vi "Add Boost Stage.vi"(8 "error in (no error)":errorcluster, 10 "Stage Name":string, 11 "Shot Section Item Ref":T1=18446744073709551615 format="%.0x") -> (0 "error out":errorcluster, 3 "Shot Section Item Ref dup":T1=18446744073709551615 format="%.0x")   [LabVIEW 2019, in "Fuel Injector Analysis Addon System Explorer.lvlib"]
uses:
  Fuel Injector Analysis Addon System Explorer.lvlib
  <vilib>/NI VeriStand/Custom Device API/Custom Device Item Ref.ctl
  Addon Shared/Types/Analysis.Channels.Select.ctl
  Addon Shared/Constants.vi
  Addon Shared/Fuel Injector Analysis Addon Shared.lvlib
  <vilib>/NI VeriStand/Custom Device API/Custom Device API.lvlib
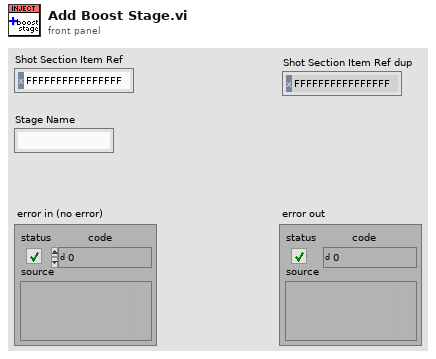
[diagram p1: front panel]
types:
  T1 = typedef "Custom Device API.lvlib/Custom Device Item Ref.ctl" = u64
  T2 = typedef "Fuel Injector Analysis Addon Shared.lvlib/Analysis.Channels.Select.ctl" = cluster{"Pull In Time":bool, "Pull In Max Current":bool, "Pull In Max Voltage":bool, "Pull In Min Voltage":bool, "Pull In Avg Voltage":bool, "Hold Time":bool, "Hold Max Current":bool, "Hold Min Current":bool, "Hold Avg Current":bool, "Hold Max Voltage":bool, "Hold Min Voltage":bool, "Hold Avg Max Voltage":bool, "Hold Avg Min Voltage":bool, "Off Time":bool, "Off Max Current":bool, "Off Min Current":bool, "Off Avg Current":bool, "Off Max Voltage":bool, "Off Min Voltage":bool, "Off Avg Voltage":bool, "Total Voltage Pulses":bool, "Total Stage Time":bool}
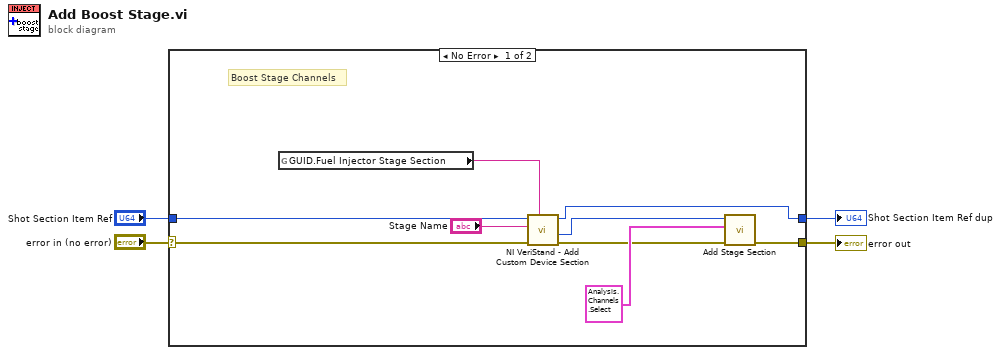
[diagram p0: block diagram]
diagram:
  n1 = case shown="No Error" "error in (no error)" {
    selector: "error in (no error)" -> [w11 w14]
    tunnel: "Shot Section Item Ref" -> [w10 w15]
    tunnel: [w5 w15] -> w2
    tunnel: [w13 w14] -> w1
    frame No Error {
      # "Boost Stage Channels"
      n2 = global read "Constants.vi" "GUID.Fuel Injector Stage Section"() -> (w12:string)
      n3 = call <vilib>:"NI VeriStand - Add Custom Device Section.vi"("GUID (Default Section)"=w12, "error in (no error)"=w11, "Section Name"="Stage Name", "Parent Ref in"=w10) -> ("error out"=w7:errorcluster, "Section Ptr"=w6:T1, "Parent Ref out"=w5:T1)  [unwired: 4 in, 1 out]
      n4 = call "Add Stage Section.vi"("error in (no error)"=w7, "Analysis Options"=T2 {"Pull In Time"=TRUE, "Pull In Max Current"=TRUE, "Pull In Max Voltage"=TRUE, "Pull In Min Voltage"=TRUE, "Pull In Avg Voltage"=TRUE, "Hold Time"=TRUE, "Hold Max Current"=TRUE, "Hold Min Current"=TRUE, "Hold Avg Current"=TRUE, "Hold Max Voltage"=TRUE, "Hold Min Voltage"=TRUE, "Hold Avg Max Voltage"=TRUE, "Hold Avg Min Voltage"=TRUE, "Off Time"=TRUE, "Off Max Current"=TRUE, "Off Min Current"=TRUE, "Off Avg Current"=TRUE, "Off Max Voltage"=TRUE, "Off Min Voltage"=TRUE, "Off Avg Voltage"=TRUE, "Total Voltage Pulses"=TRUE, "Total Stage Time"=TRUE}, "Shot Section reference in"=w6) -> ("error out"=w13:errorcluster)  [unwired: 7 in, 1 out]
    }
    frame Error {
    }
  }
  "error out" <- w1
  "Shot Section Item Ref dup" <- w2
